vi "PassObserverTactic.vi"(1 "Game in":refnum<class "Game.lvclass">, 8 "error in (no error)":errorcluster, 9 "first call":bool, 10 "Robot":refnum<class "Robot.lvclass">, 11 "PassObserverTactic in":refnum<class "PassObserverTactic.lvclass">) -> (0 "error out":errorcluster, 2 "Robot":refnum<class "Robot.lvclass">, 3 "PassObserverTactic out":refnum<class "PassObserverTactic.lvclass">)   [LabVIEW 2020, in "PassObserverTactic.lvclass"]
uses:
  PassObserverTactic.lvclass
  Robot_class/Robot.lvclass
  Game_class/Game.lvclass
  Robot_class/tactics.ctl
  Tactic_class/Tactic.lvclass/Tactic.ctl
  Robot_class/Robot.lvclass/Robot.ctl
  Tactic_class/Read Skillbook.vi
  Robot_class/Write tactic.vi
  Skillbook_class/Skillbook.lvclass
  PassObserverSkill_class/PassObserverSkill.lvclass
panel:
  out "x .or. y?":bool
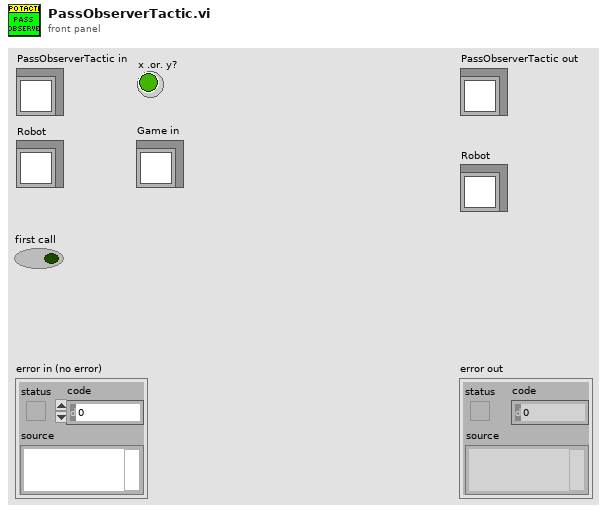
[diagram p1: front panel]
types:
  T1 = typedef "tactics.ctl" = enum16{"PenaltyAttacker", "DefaultPs", "PassObserver", "PenaltyDefense", "Test", "DefendGoal", "Marker", "FollowAttacker", "DefendArea", "Shoot", "AttackerAimGoal", "AttackerBallOutOfField", "AttackerBlock", "AttackerStop", "Duelist", "Halt", "ZigZag", "GoTo", "Timeout", "KickToPassReceiver", "PositionToReceivePass", "PassReceiver", "WaitPass"}
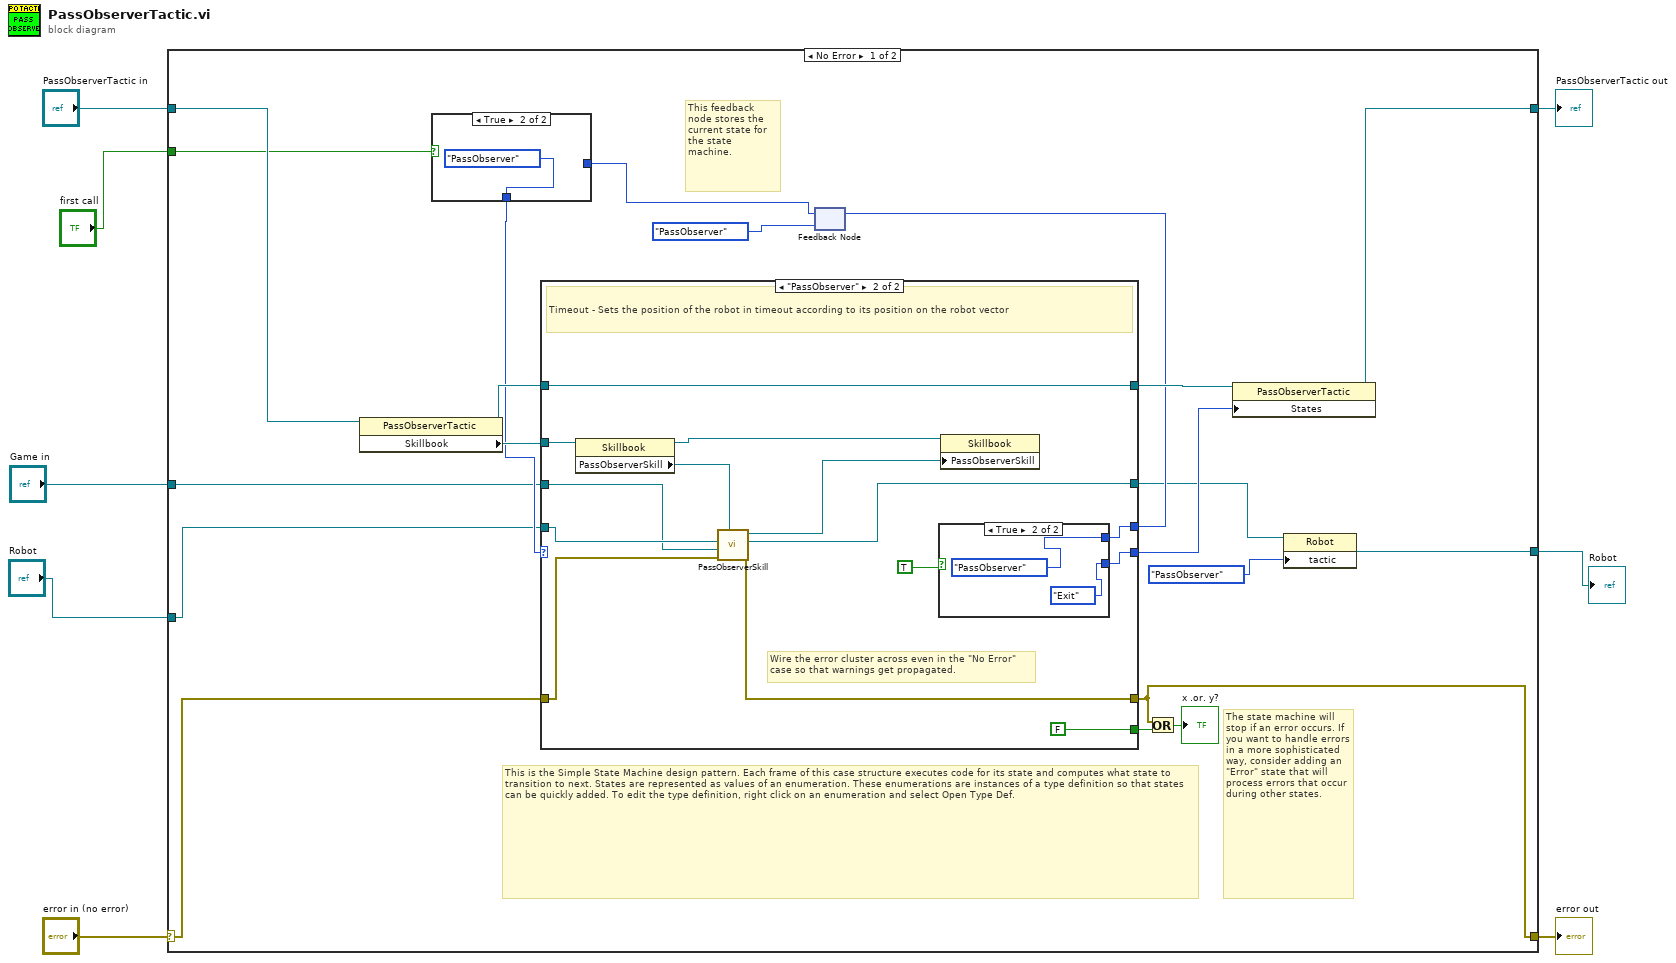
[diagram p0: block diagram]
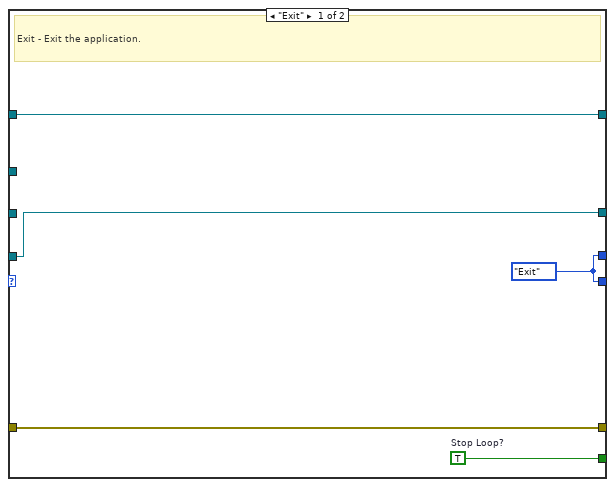
[diagram p3: hidden frame]
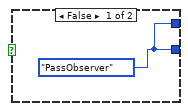
[diagram p4: hidden frame]
diagram:
  n1 = case shown="No Error" "error in (no error)" {
    selector: "error in (no error)" -> [w17 w55]
    tunnel: [w16 w55] -> w7
    tunnel: [w13 w54] -> w5
    tunnel: "PassObserverTactic in" -> [w14 w54]
    tunnel: "Robot" -> [w11 w53]
    tunnel: [w15 w53] -> w3
    tunnel: "first call" -> [w10 _]
    tunnel: "Game in" -> [w9 _]
    frame No Error {
      # "The state machine will stop if an error occurs. If you want to handle errors in a more sophisticated way, consider adding an \"Error\" state that will process errors that occur during other states."
      # "This feedback node stores the current state for the state machine."
      # "This is the Simple State Machine design pattern. Each frame of this case structure executes code for its state and computes what state to transition to next. States are represented as values of an enumeration. These enumerations are instances of a type definition so that states can be quickly added. To edit the type definition, right click on an enumeration and select Open Type Def."
      # "Wire the error cluster across even in the \"No Error\"\ncase so that warnings get propagated."
      n2 = property class="PassObserverTactic"(reference=w14) -> (reference out=w24:refnum<class "PassObserverTactic.lvclass">, "Skillbook"=w26:refnum<class "Skillbook.lvclass">)  [unwired: 1 in, 1 out]
      n3 = feedback #1(enum16{"PassObserver", "Exit"}."PassObserver" ("States")) -> (w20:enum16{"PassObserver", "Exit"})
      n4 = case shown="True" w10 {
        tunnel: [w29 enum16{"PassObserver", "Exit"}."PassObserver" ("States")] -> w21
        tunnel: w20 -> [w29 _]
        frame False {
        }
        frame True {
        }
      }
      n5 = case shown="\"PassObserver\"" w21 {
        tunnel: [w31 w46] -> w23
        tunnel: [w35 FALSE ("Stop Loop?")] -> w28
        tunnel: w17 -> [w34 w39]
        tunnel: [w34 w38] -> w16
        tunnel: w26 -> [_ w48]
        tunnel: w11 -> [w33 w40]
        tunnel: [w33 w41] -> w18
        tunnel: [w32 w47] -> w25
        tunnel: w24 -> [w32 w47]
        tunnel: [w31 w45] -> w22
        tunnel: w9 -> [_ w37]
        frame "Exit" {
          w31 = enum16{"PassObserver", "Exit"}."Exit" ("States")
          w35 = TRUE  # Stop Loop?
          # "Exit - Exit the application."
        }
        frame "PassObserver" {
          # "Timeout - Sets the position of the robot in timeout according to its position on the robot vector"
          n6 = property class="Skillbook"(reference=w48) -> (reference out=w43:refnum<class "Skillbook.lvclass">, "PassObserverSkill"=w44:refnum<class "PassObserverSkill.lvclass">)  [unwired: 1 in, 1 out]
          n7 = call-dynamic "PassObserverSkill.vi"("error in (no error)"=w39, "Game in"=w37, "Robot"=w40, "PassObserverSkill in"=w44) -> ("error out"=w38:errorcluster, "Robot"=w41:refnum<class "Robot.lvclass">, "PassObserverSkill out"=w42:refnum<class "PassObserverSkill.lvclass">)  [unwired: 4 in, 1 out]
          n8 = case shown="True" TRUE {
            tunnel: [w50 enum16{"PassObserver", "Exit"}."Exit" ("States")] -> w46
            tunnel: [w50 enum16{"PassObserver", "Exit"}."PassObserver" ("States")] -> w45
            frame False {
              w50 = enum16{"PassObserver", "Exit"}."PassObserver" ("States")
            }
            frame True {
            }
          }
          n9 = property class="Skillbook"(reference=w43, "PassObserverSkill"=w42) -> ()  [unwired: 1 in, 2 out]
        }
      }
      n10 = feedback-in #1(w22) -> ()
      n11 = Or(x=w16, y=w28) -> (x .or. y?=→"x .or. y?":bool)
      n12 = property class="PassObserverTactic"(reference=w25, "States"=w23) -> (reference out=w13:refnum<class "PassObserverTactic.lvclass">)  [unwired: 1 in, 1 out]
      n13 = property class="Robot"(reference=w18, "tactic"=tactics."PassObserver") -> (reference out=w15:refnum<class "Robot.lvclass">)  [unwired: 1 in, 1 out]
    }
    frame Error {
      # "Wire the error cluster across even in the \"No Error\"\ncase so that warnings get propagated."
    }
  }
  "error out" <- w7
  "PassObserverTactic out" <- w5
  "Robot" <- w3
